vi "write_device_object_sdo.vi"(0 "node":u8, 5 "index":u16, 7 "subind":u8, 9 "data":u8[](array[numeric]), 11 "datasize":u32) -> (4 "return":i16)   [LabVIEW 2011]
uses:
  canopen_dll_master.dll
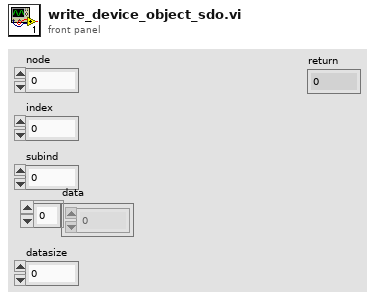
[diagram p1: front panel]
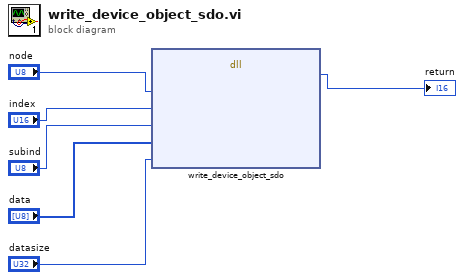
[diagram p0: block diagram]
diagram:
  n1 = dll-call lib="canopen_dll_master.dll" fn="write_device_object_sdo"("node"="node", "index"="index", "subind"="subind", "data"="data", "datasize"="datasize") -> ("return type"=→"return":i16)  [unwired: 8 in, 2 out]
